vi "Authenticate Core.vi"(8 "error in (no error)":errorcluster, 9 "Password":string, 10 "Username":string, 11 "LDAP Authentication in":refnum<class "LDAP Authentication.lvclass">) -> (0 "error out":errorcluster, 2 "Authenticated?":bool, 3 "LDAP Authentication out":refnum<class "LDAP Authentication.lvclass">)   [LabVIEW 2016, in "LDAP Authentication.lvclass"]
uses:
  LDAP Authentication.lvclass
  LDAP Authentication.lvclass/LDAP Authentication.ctl
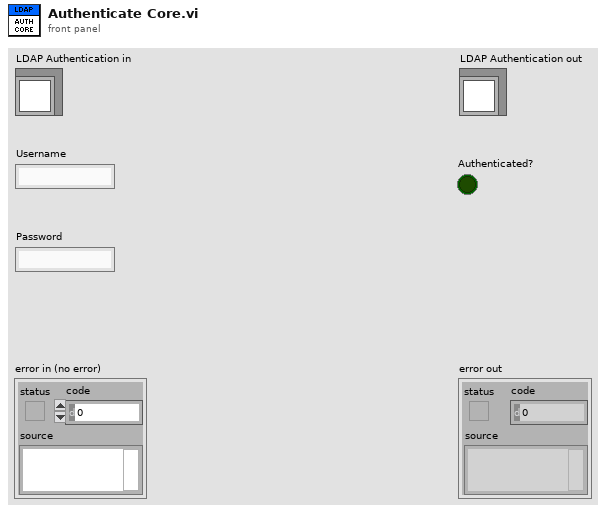
[diagram p1: front panel]
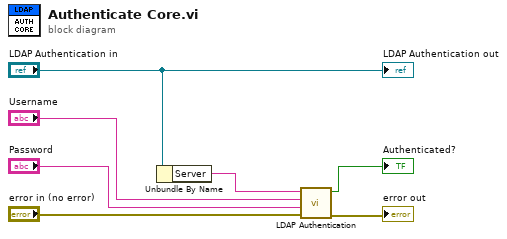
[diagram p0: block diagram]
diagram:
  n1 = Unbundle By Name("LDAP Authentication in") -> ("Server"=w1:string)
  n2 = call "LDAP Authentication.vi"("error in (no error)"="error in (no error)", "Password"="Password", "User Name"="Username", "Server"=w1) -> ("error out"=→"error out":errorcluster, "Valid?"=→"Authenticated?":bool)  [unwired: 6 in]
  "LDAP Authentication out" <- "LDAP Authentication in"
